vi "read_xy_ADC.vi"(7 "x(0), y(0)":fxp<+/-,16,5>[](array[numeric]), 10 "y - ADC":refnum<k21>="Mod2/AI1", 11 "x - ADC":refnum<k21>="Mod2/AI0") -> (2 "x_y":fxp<+/-,17,6>[](array[numeric]))   [LabVIEW 2017]
uses:
  <vilib>/rvi/eio/common/nirviEmuTemplateMethod_errors.vi
  <vilib>/eio/EIONode/EIONode.xnode
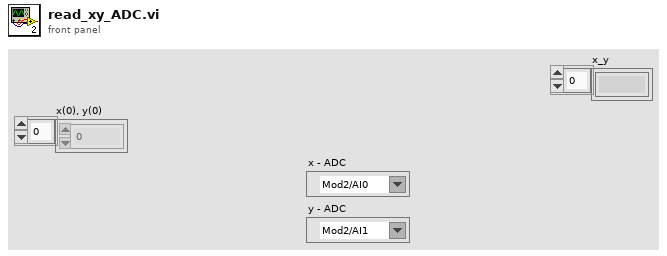
[diagram p1: front panel]
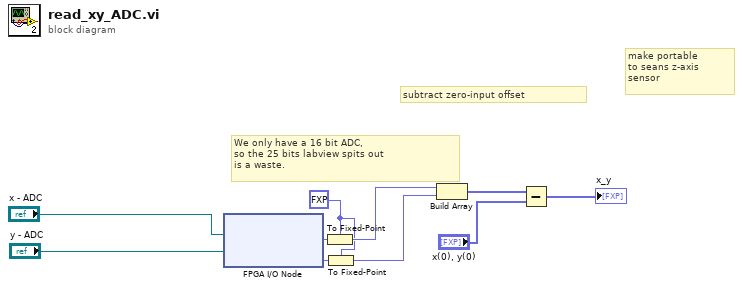
[diagram p0: block diagram]
diagram:
  w2 = fxp<+/-,16,5> 0.0 ("fixed-point type")
  # "We only have a 16 bit ADC,\nso the 25 bits labview spits out\nis a waste."
  # "make portable\nto seans z-axis\nsensor"
  # "subtract zero-input offset"
  n1 = xnode "FPGA I/O Node"("FPGA I/O In"="x - ADC", "FPGA I/O In"="y - ADC") -> ("I/O Item"=w6:fxp<+/-,24,5>, "I/O Item"=w4:fxp<+/-,24,5>)  [unwired: 2 out]
  n2 = To Fixed-Point(fixed-point type=w2, number=w6) -> (fixed-point=w5:fxp<+/-,16,5>)
  n3 = To Fixed-Point(fixed-point type=w2, number=w4) -> (fixed-point=w3:fxp<+/-,16,5>)
  n4 = Build Array(w5, w3) -> (w10:fxp<+/-,16,5>[])
  n5 = Subtract(x=w10, y="x(0), y(0)") -> (x-y=→"x_y":fxp<+/-,17,6>[])
